vi "CalcDist2Circle.vi"(2 "X-cords":dbl, 3 "Height of circle":dbl=10.0) -> (0 "Angle to circle":dbl, 1 "Distance":dbl)   [LabVIEW 2009, in "ImageAnalysis.lvlib"]
uses:
  ImageAnalysis.lvlib
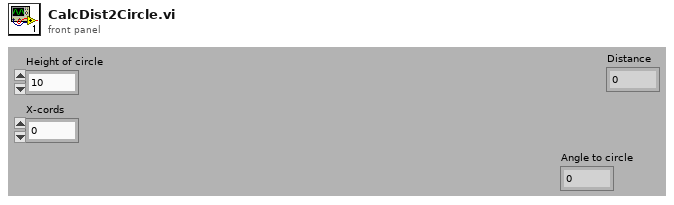
[diagram p1: front panel]
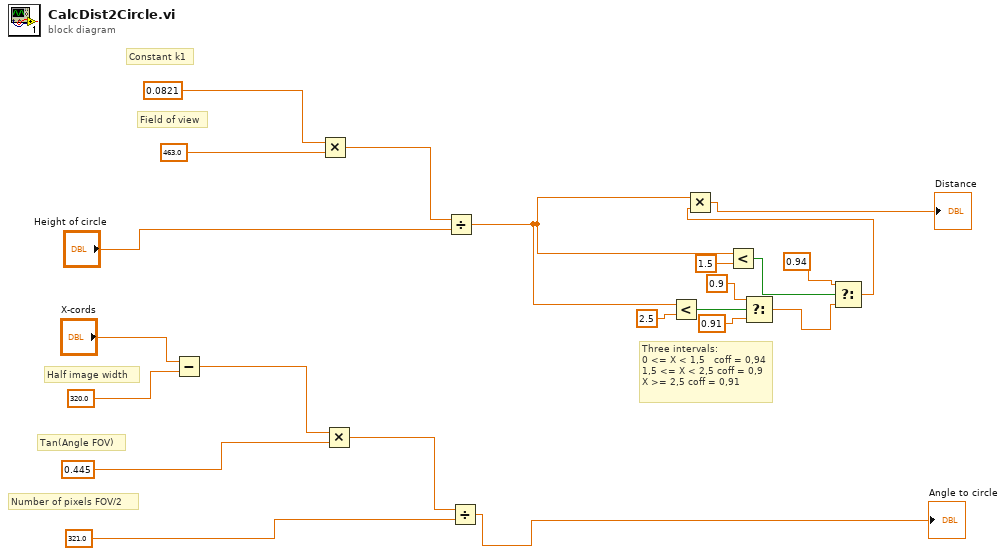
[diagram p0: block diagram]
diagram:
  # "Three intervals:\n0 <= X < 1,5   coff = 0,94\n1,5 <= X < 2,5 coff = 0,9\nX >= 2,5 coff = 0,91"
  # "Half image width"
  # "Number of pixels FOV/2"
  # "Tan(Angle FOV)"
  # "Constant k1"
  # "Field of view"
  n1 = Subtract(x="X-cords", y=320.0) -> (x-y=w14:dbl)
  n2 = Multiply(x=0.0821, y=463.0) -> (x*y=w21:dbl)
  n3 = Multiply(x=w14, y=0.445) -> (x*y=w19:dbl)
  n4 = Divide(x=w21, y="Height of circle") -> (x/y=w2:dbl)
  n5 = Divide(x=w19, y=321.0) -> (x/y=→"Angle to circle":dbl)
  n6 = Less?(x=w2, y=2.5) -> (x < y?=w10:bool)
  n7 = Less?(x=w2, y=1.5) -> (x < y?=w4:bool)
  n8 = Select(t=0.9, s=w10, f=0.91) -> (s? t:f=w6:dbl)
  n9 = Select(t=0.94 ("f"), s=w4, f=w6) -> (s? t:f=w1:dbl)
  n10 = Multiply(x=w2, y=w1) -> (x*y=→"Distance":dbl)
